vi "Get VISA Resource.vi"(8 "error in (no error)":errorcluster, 11 "EPU452 in":refnum<class "EPU452.lvclass">) -> (0 "error out":errorcluster, 2 "VISA Resource":refnum<visa-resource-name>, 3 "EPU452 out":refnum<class "EPU452.lvclass">)   [LabVIEW 2018, in "EPU452.lvclass"]
uses:
  EPU452.lvclass
  EPU452.lvclass/EPU452.ctl
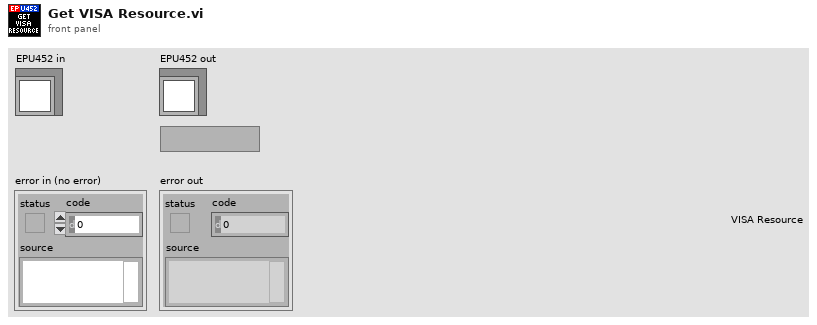
[diagram p1: front panel]
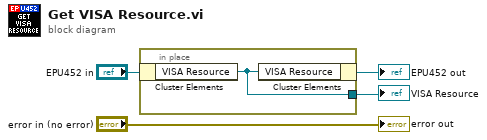
[diagram p0: block diagram]
diagram:
  n1 = in-place {
    in-place-border: [w5] -> w2
    n2 = in-place-cluster #1("EPU452 in") -> ("VISA Resource"=w5:refnum<visa-resource-name>)
    n3 = in-place-cluster #1("VISA Resource"=w5) -> (→"EPU452 out":refnum<class "EPU452.lvclass">)
  }
  "VISA Resource" <- w2
  "error out" <- "error in (no error)"
